vi "USBImageContinuousV1.4.vi"() -> ()   [LabVIEW 2017]
uses:
  C:/Program Files (x86)/National Instruments/LabVIEW 2019/ATMCD32D.dll
  <vilib>/Utility/file.llb/Write Delimited Spreadsheet (I64).vi
  C:/Users/Spenser Burrows/Desktop/Work/Labview software for spectrometer/PiezoStage_John/Piezojena.Protocols.Nv40Single.dll
  E/PiezoStage_John/piezojena NV40Single.lvlib
panel:
  in  "Tab Control":T1(tab)
  out "Expected position on spectrometer (pixels):":dbl
  in  "Harmonic":dbl min=10.0 max=40.0
  out "l (nm)":dbl
  out "E (J)":dbl
  out "E (eV)":dbl
  out "Nearest Harmonic of 800nm":dbl
  out "Cursor Position (pixels)":dbl
  out "Distance to nearest harmonic of 800nm (pixels)":dbl
  in  "Grating:":u16(ring) items=["Shimadzu 30-006  "]
  in  "Laser:":u16(ring) items=["800nm  "]
  in  "Trigger":u32(ring) items=["Internal", "External"]
  out "Initialize":u32
  in  "Exposure Time (secs)":sgl format="%.2f"
  out "Calculated Exposure Value":sgl format="%.5f"
  out "Get Acquired Data":u32
  out "Start Acquisition":u32
  out "Detector X Pixels":i32
  out "Check Timings":u32
  out "Set Acquisition Mode":u32
  out "Set Readout Mode":u32
  out "Set Trigger Mode":u32
  out "Set Exposure Time":u32
  out "Get Detector":u32
  out "Detector Y Pixels":i32
  out "Shut Down":u32
  out "Set Gate Mode":u32
  out "Set Image":u32
  out "Raw Image From Camera":i32[][](graph)
  out "Vertical Binned Waveform Graph":i32[](graph)
  out "Get Status":u32
  in  "Stop":bool
  in  "Save image":bool
  out "Camera Status:":bool
  out "Last Image Saved:":string
  in  "Caibration Date":u16(ring) items=["first calibration - 7/31", "7/31-current"]
  out "Wavelength Graph (nm)":cluster{"No prefix":dbl, i32}[](graph)
  out "Energy Graph (eV)":cluster{"eV":dbl, i32}[](graph)
  out "Harmonics Graph":cluster{"No prefix":dbl, i32}[](graph)
  in  "Measurement Length [fs]":ext=30.0
  out "Optical Cycles \nin measurement":ext=16.905589736842103296
  in  "Initial Piezo Position":sgl=40.0
  out "Number of Steps":ext=300.00000000000005795
  in  "Step Size [as]":sgl=100.0
  in  "?":bool
  in  "Settings":bool
  in  "Wavelength (nm)":i32(listbox)
  in  "Piezojena Seriel Port":refnum<visa-resource-name>="COM4"
  out "Piezo Voltage Supply":cluster{dbl[], dbl[]}(graph)={[0.0], [70.08999633789062]}
  in  "Initial Piezo Position [um]":dbl(slide)=40.0 scale=0.0..80.0
  in  "Final Piezo Position [um]":dbl(slide)=48.99377374 scale=0.0..80.0
  out "Volt Meter":dbl(knob)=70.08999633789062 scale=-10.0..150.0
  out "Raw Image From Camera":i32[][](graph)
  out "Status":u32
  # "Status"
  # "Return values"
  # "Acquisition Mode: Single Scan\nReadout Mode: Full Resolution Image"
  # "XUV Spectrometer Control VI"
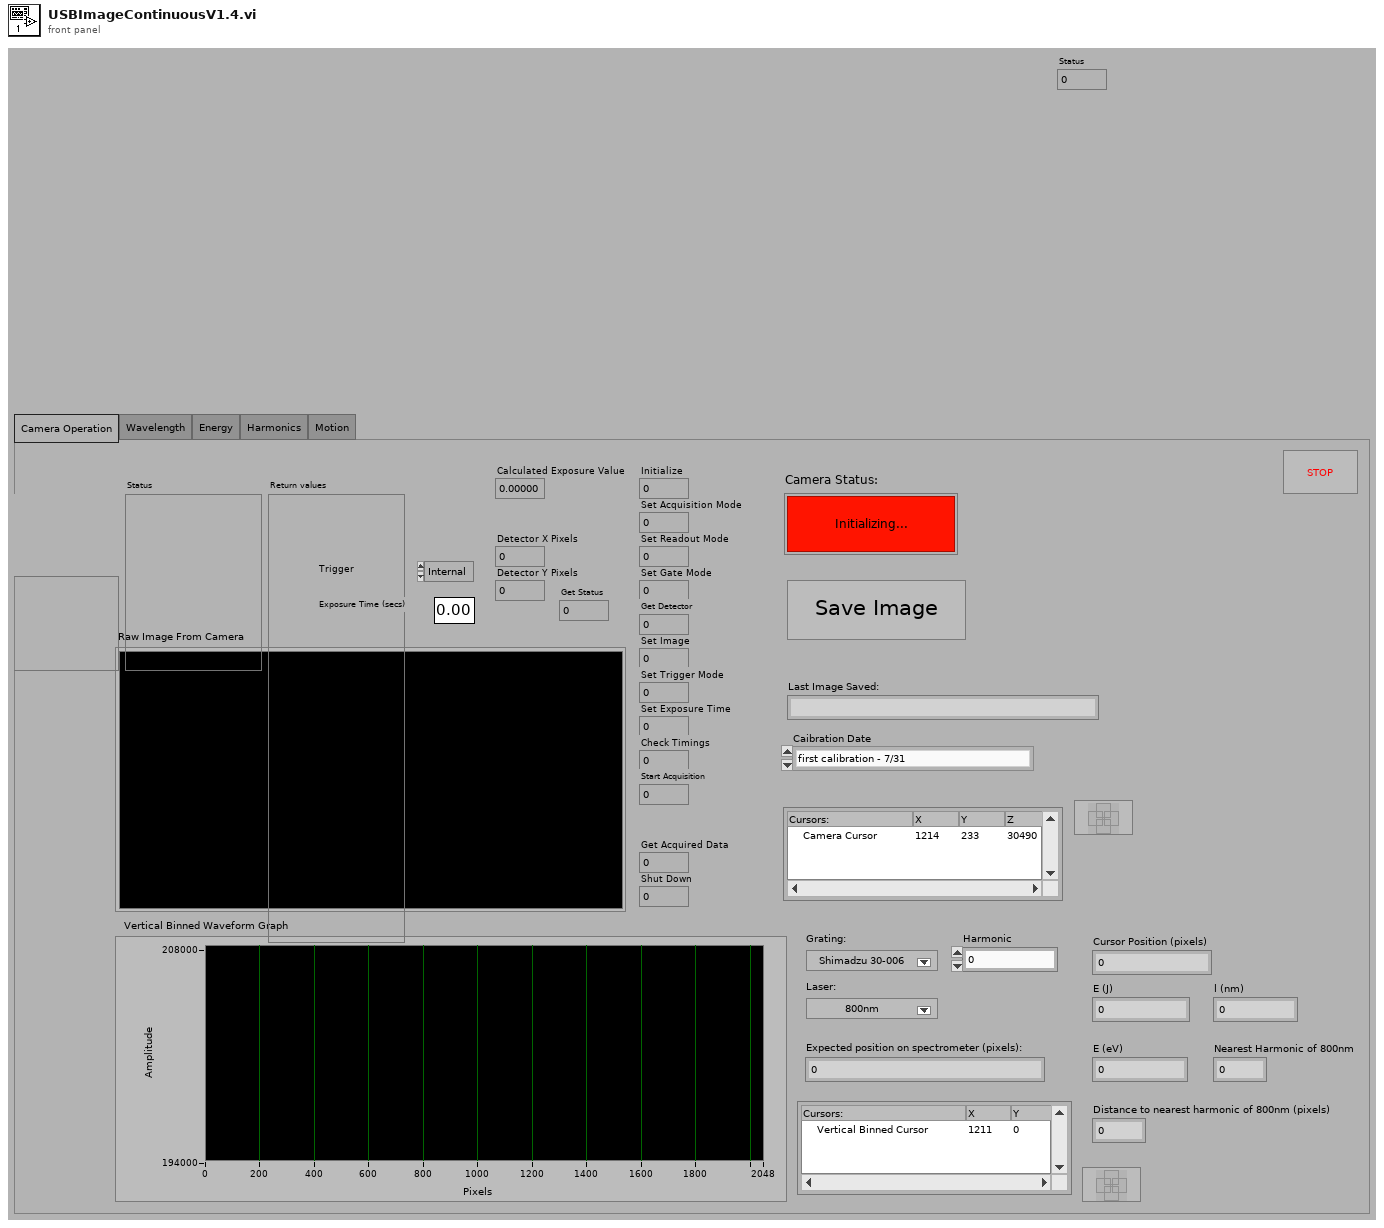
[diagram p1: front panel]
types:
  T1 = enum32{"Camera Operation", "Wavelength", "Energy", "Harmonics", "Motion"}
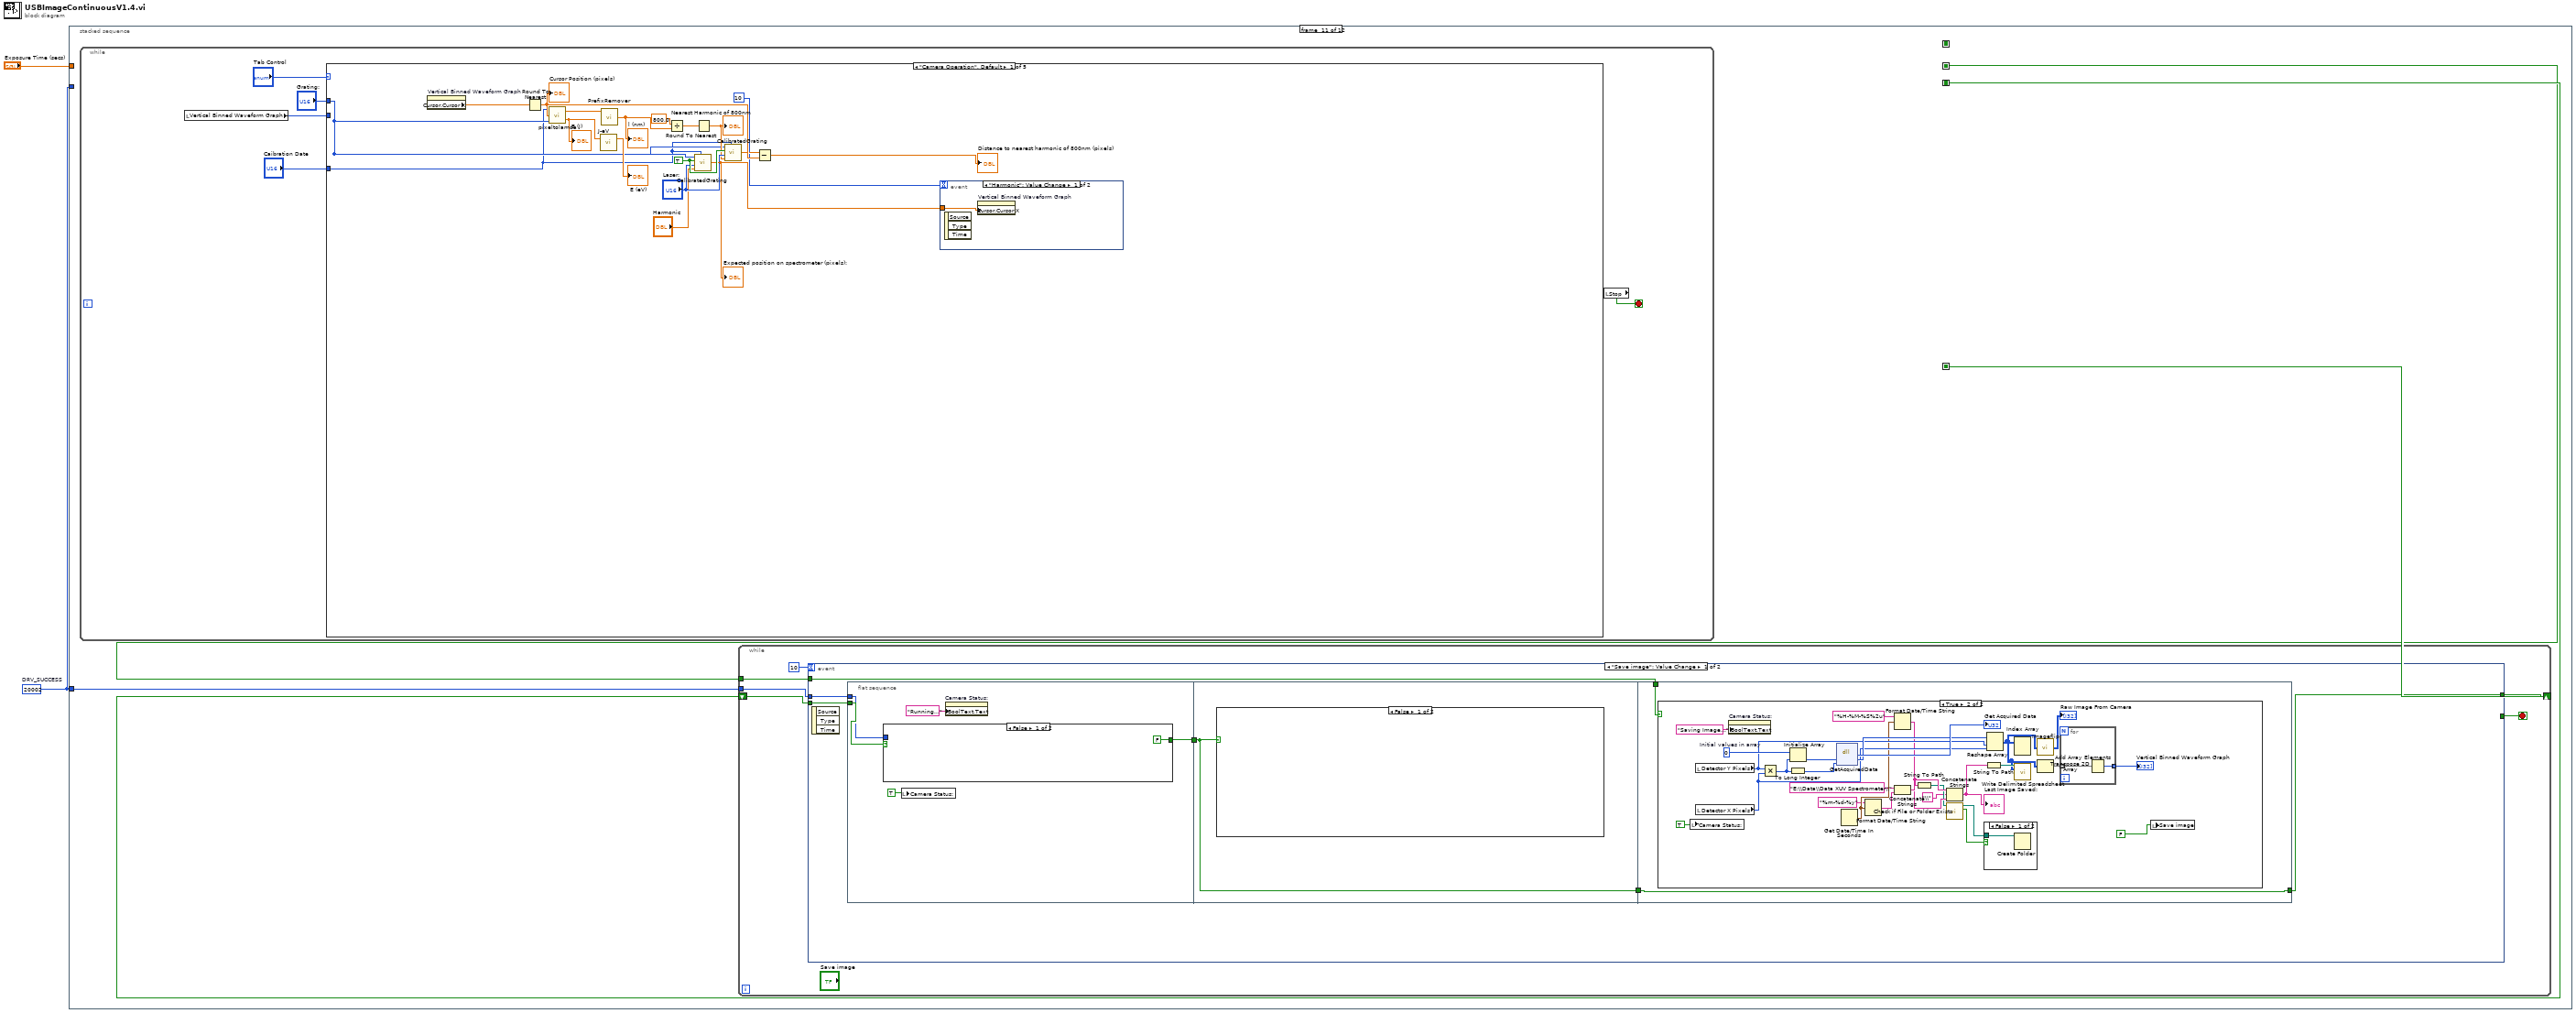
[diagram p0: block diagram]
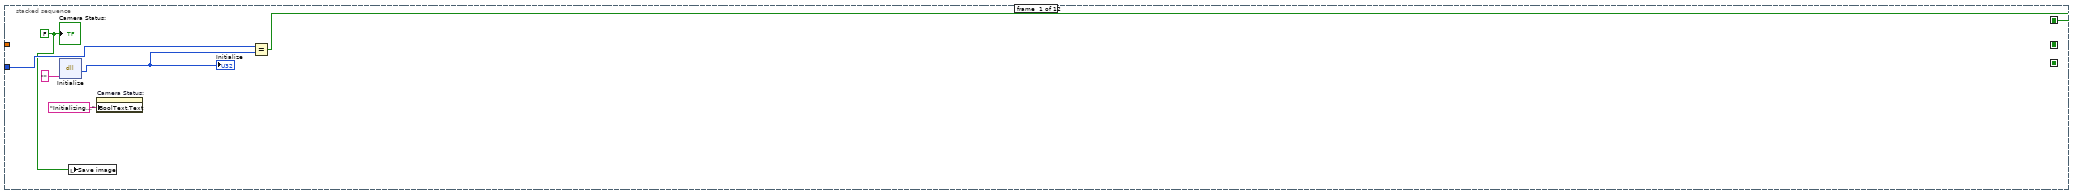
[diagram p2: hidden frame]
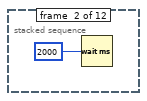
[diagram p3: hidden frame]
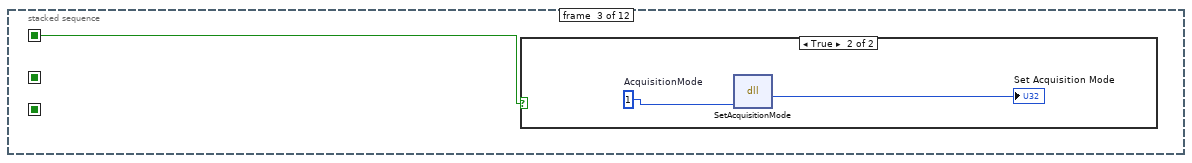
[diagram p4: hidden frame]
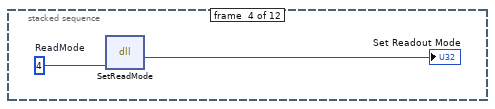
[diagram p6: hidden frame]
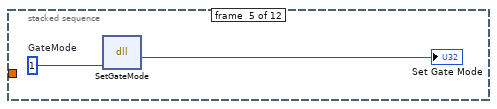
[diagram p7: hidden frame]
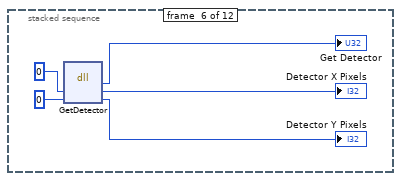
[diagram p8: hidden frame]
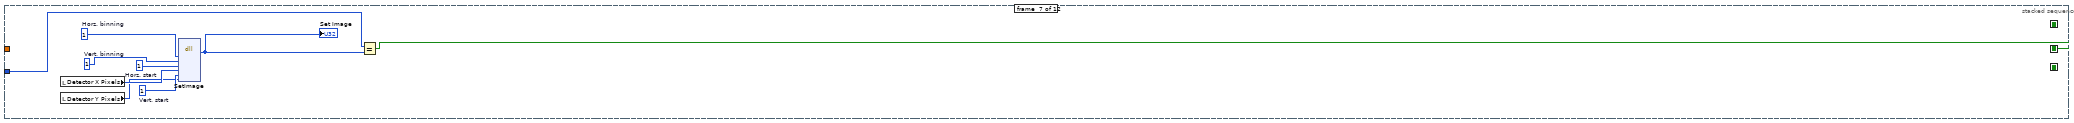
[diagram p9: hidden frame]
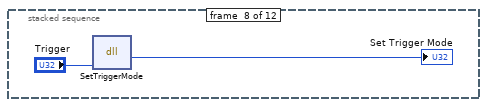
[diagram p10: hidden frame]
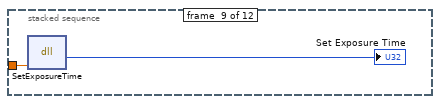
[diagram p11: hidden frame]
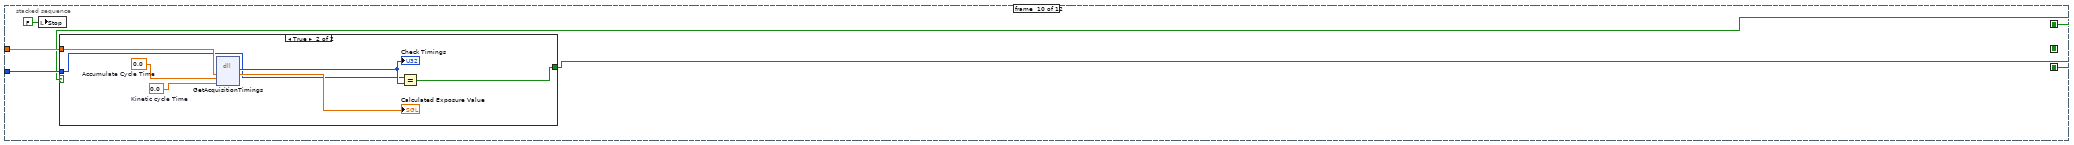
[diagram p12: hidden frame]
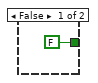
[diagram p13: hidden frame]
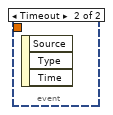
[diagram p14: hidden frame]
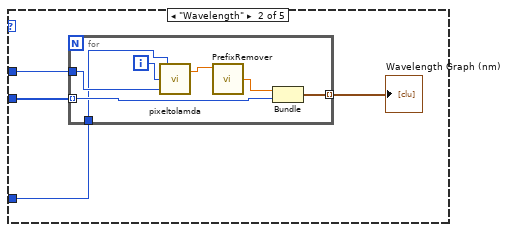
[diagram p15: hidden frame]
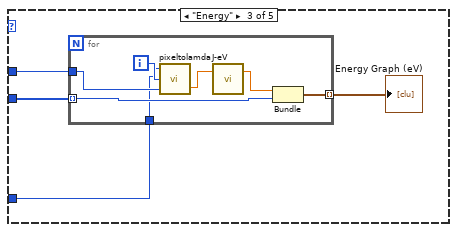
[diagram p16: hidden frame]
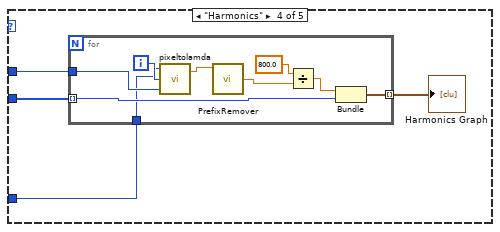
[diagram p17: hidden frame]
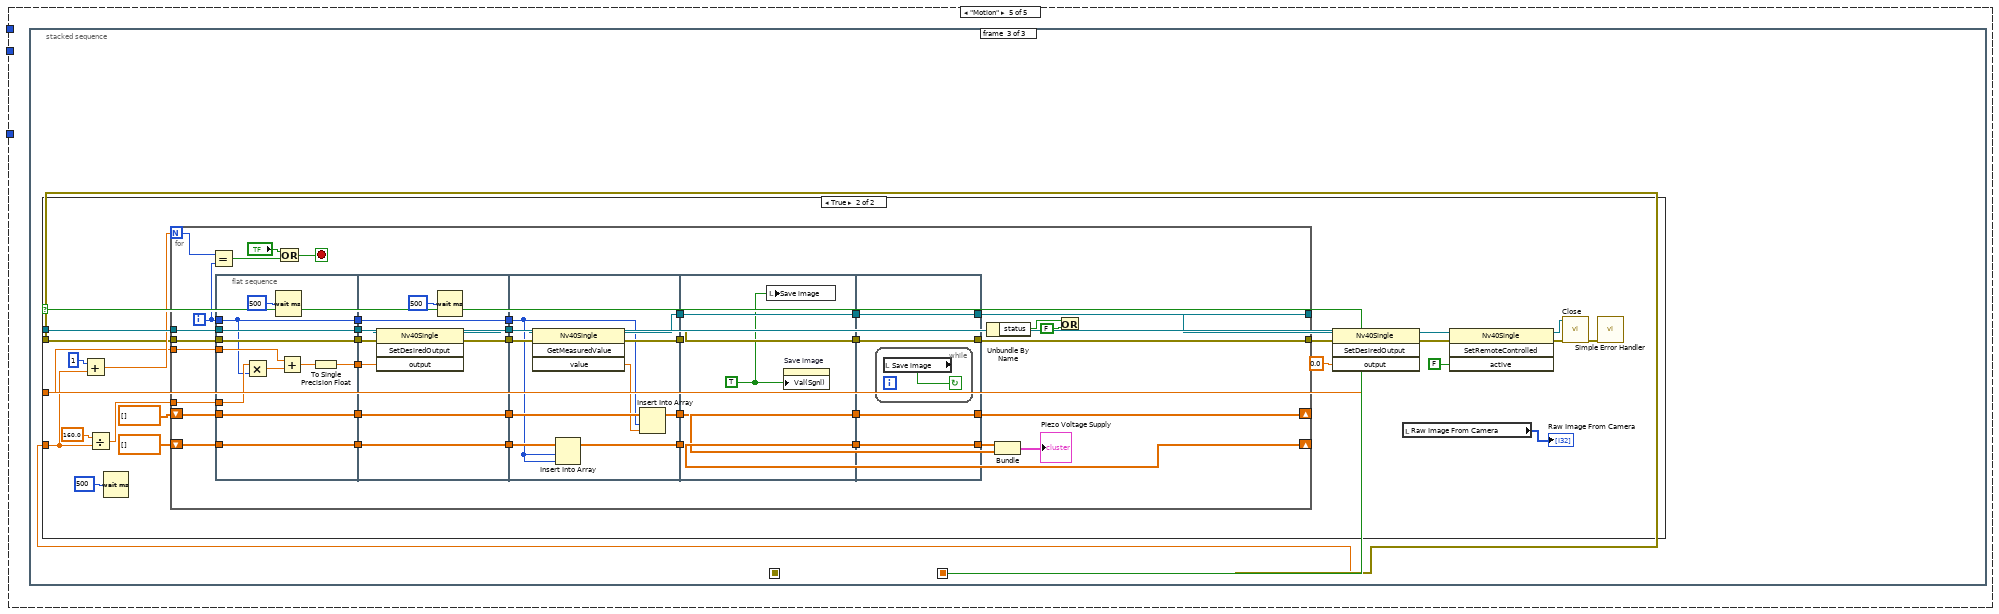
[diagram p18: hidden frame]
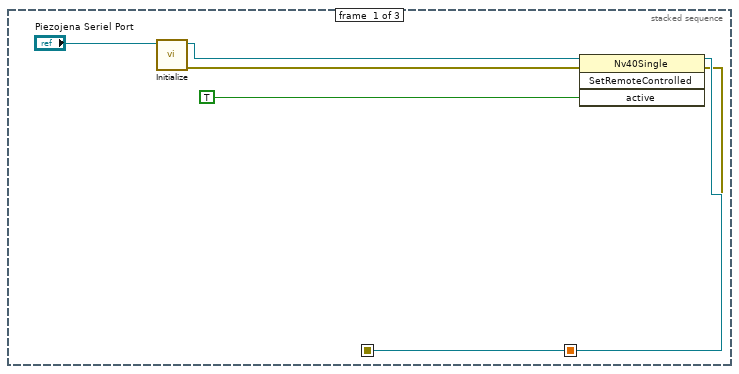
[diagram p19: hidden frame]
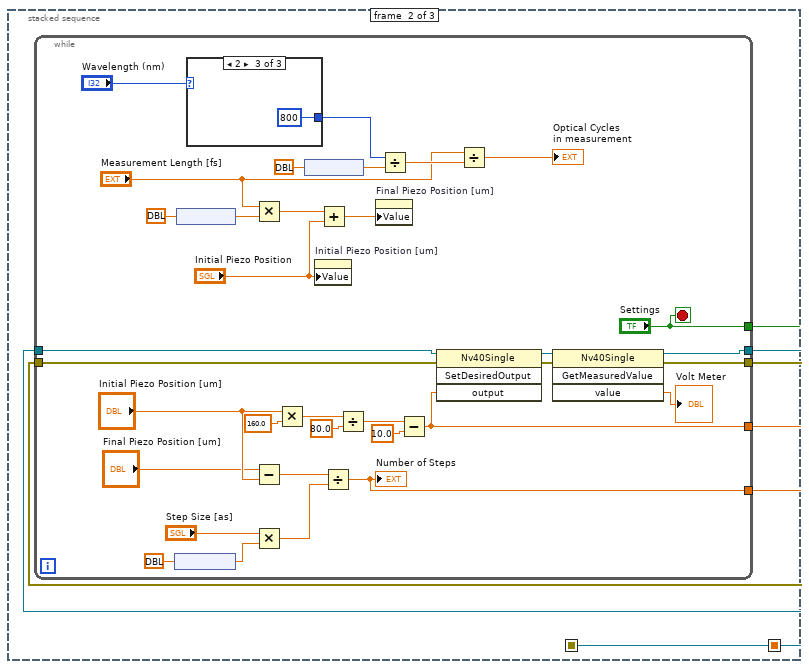
[diagram p20: hidden frame]
diagram:
  w1 = 20002  # DRV_SUCCESS
  n1 = stacked-sequence {
    seq-local: [w6 _ _ _ _ _ _ _ _ _ _ _] -> [_ _ w10 _ _ _ _ _ _ w36 _ w378]
    seq-local: [_ _ _ _ _ _ _ _ _ w37 _ _] -> [_ _ _ _ _ _ _ _ _ _ w51 _]
    seq-local: [_ _ _ _ _ _ _ _ _ _ w49 _] -> [_ _ _ _ _ _ _ _ _ _ _ _]
    seq-local: [_ _ _ _ _ _ w22 _ _ _ _ _] -> [_ _ _ _ _ _ _ _ _ _ w48 _]
    tunnel: "Exposure Time (secs)" -> [_ _ _ _ _ _ _ _ w34 w39 _ _]
    tunnel: w1 -> [w7 _ _ _ _ _ w24 _ _ w38 _ _]
    tunnel: w1 -> [_ _ _ _ _ _ _ _ _ _ w50 _]
    frame #0 {
      w3 = FALSE ("Camera Status:")
      n2 = dll-call lib="C:/Program Files (x86)/National Instruments/LabVIEW 2019/atmcd32d.dll" fn="Initialize" label="Call Library Function Initialize"("") -> (w8:u32)  [unwired: 4 in, 2 out]
      "Initialize" <- w8
      n3 = local write "Save image"(w3) -> ()
      n4 = property on="Camera Status:" class="Bool (strict)"("BoolText.Text"="Initializing..." ("String")) -> ()  [unwired: 2 in, 2 out]
      n5 = Equal?(x=w7, y=w8) -> (x = y?=w6:bool)
      "Camera Status:" <- w3
    }
    frame #1 {
      n6 = Wait (ms)(milliseconds to wait=u32 2000) -> ()  [unwired: 1 out]
    }
    frame #2 {
      n7 = case shown="True" w10 {
        frame False {
        }
        frame True {
          w12 = u16 1  # AcquisitionMode
          n8 = dll-call lib="C:/Program Files (x86)/National Instruments/LabVIEW 2019/atmcd32d.dll" fn="SetAcquisitionMode" label="Call Library Function SetAcquisitionMode"(w12) -> (→"Set Acquisition Mode":u32)  [unwired: 4 in, 2 out]
        }
      }
    }
    frame #3 {
      w14 = u16 4  # ReadMode
      n9 = dll-call lib="C:/Program Files (x86)/National Instruments/LabVIEW 2019/atmcd32d.dll" fn="SetReadMode" label="Call Library Function SetReadMode"(w14) -> (→"Set Readout Mode":u32)  [unwired: 4 in, 2 out]
    }
    frame #4 {
      w16 = u16 1  # GateMode
      n10 = dll-call lib="C:/Program Files (x86)/National Instruments/LabVIEW 2019/atmcd32d.dll" fn="SetGateMode" label="Call Library Function SetGateMode"(w16) -> (→"Set Gate Mode":u32)  [unwired: 4 in, 2 out]
    }
    frame #5 {
      n11 = dll-call lib="C:/Program Files (x86)/National Instruments/LabVIEW 2019/atmcd32d.dll" fn="GetDetector" label="Call Library FunctionGetDetector"(i16 0, i16 0) -> (→"Get Detector":u32, →"Detector X Pixels":i32, →"Detector Y Pixels":i32)  [unwired: 3 in, 2 out]
    }
    frame #6 {
      w27 = u16 1  # Vert. start
      w28 = u16 1  # Horz. start
      w29 = u16 1  # Vert. binning
      w30 = u16 1  # Horz. binning
      n12 = local read "Detector X Pixels"() -> (w26:i32)
      n13 = local read "Detector Y Pixels"() -> (w25:i32)
      n14 = dll-call lib="C:/Program Files (x86)/National Instruments/LabVIEW 2019/atmcd32d.dll" fn="SetImage" label="Call Library Function SetImage"(w30, w29, w28, w26, w27, w25) -> (w23:u32)  [unwired: 9 in, 2 out]
      "Set Image" <- w23
      n15 = Equal?(x=w24, y=w23) -> (x = y?=w22:bool)
    }
    frame #7 {
      n16 = dll-call lib="C:/Program Files (x86)/National Instruments/LabVIEW 2019/atmcd32d.dll" fn="SetTriggerMode" label="Call Library Function SetTrigger Mode"("Trigger") -> (→"Set Trigger Mode":u32)  [unwired: 4 in, 2 out]
    }
    frame #8 {
      n17 = dll-call lib="C:/Program Files (x86)/National Instruments/LabVIEW 2019/atmcd32d.dll" fn="SetExposureTime" label="Call Library FunctionSet Exposure Time"(w34) -> (→"Set Exposure Time":u32)  [unwired: 4 in, 2 out]
    }
    frame #9 {
      n18 = local write "Stop"(FALSE ("Stop")) -> ()
      n19 = case shown="True" w36 {
        tunnel: w39 -> [_ w44]
        tunnel: w38 -> [_ w41]
        tunnel: [FALSE w43] -> w37
        frame False {
        }
        frame True {
          w46 = sgl 0.0  # Accumulate Cycle Time
          w47 = sgl 0.0  # Kinetic cycle Time
          n20 = dll-call lib="C:/Program Files (x86)/National Instruments/LabVIEW 2019/atmcd32d.dll" fn="GetAcquisitionTimings" label="Call Library Function Check Timings"(w44, w46, w47) -> (w42:u32, →"Calculated Exposure Value":sgl)  [unwired: 5 in, 2 out]
          "Check Timings" <- w42
          n21 = Equal?(x=w41, y=w42) -> (x = y?=w43:bool)
        }
      }
    }
    frame #10 {
      n22 = while {
        stop <- w53 stop-if-true
        n23 = local read "Vertical Binned Waveform Graph"() -> (w55:i32[])
        n24 = case shown="\"Camera Operation\", Default" "Tab Control" {
          tunnel: w55 -> [_ w79 w90 w101 _]
          tunnel: "Grating:" -> [w58 w78 w89 w100 _]
          tunnel: "Caibration Date" -> [w57 w76 w87 w98 _]
          frame "Camera Operation", Default {
            w74 = TRUE
            n25 = property on="Vertical Binned Waveform Graph" class="WFGraph (strict)"() -> ("Cursor.Cursor X"=w71:dbl)  [unwired: 2 in, 2 out]
            n26 = Round To Nearest(number=w71) -> (nearest integer value=w64:dbl)
            "Cursor Position (pixels)" <- w64
            n27 = call "pixeltolamda.vi"("Grating:"=w58, "Pixel Postion"=w64, "Caibration Date"=w57) -> ("E (J)"=w66:dbl, "lamda (m)"=w72:dbl)
            "E (J)" <- w66
            n28 = call "J-eV.vi"("J"=w66) -> ("eV"=→"E (eV)":dbl)  [unwired: 1 in, 1 out]
            n29 = call "PrefixRemover.vi"("Nano"=w72) -> ("No prefix"=w67:dbl)  [unwired: 3 in]
            "l (nm)" <- w67
            n30 = Divide(x=800.0, y=w67) -> (x/y=w69:dbl)
            n31 = call "CalibratedGrating.vi"("Grating:"=w58, "Subvi?"=w74, "Laser:"="Laser:", "Harmonic"="Harmonic", "Caibration Date"=w57) -> ("Position on spectrometer (pixels):"=w60:dbl)
            "Expected position on spectrometer (pixels):" <- w60
            n32 = Round To Nearest(number=w69) -> (nearest integer value=w63:dbl)
            "Nearest Harmonic of 800nm" <- w63
            n33 = call "CalibratedGrating.vi"("Grating:"=w58, "Subvi?"=w74, "Laser:"="Laser:", "Harmonic"=w63, "Caibration Date"=w57) -> ("Position on spectrometer (pixels):"=w62:dbl)
            n34 = Subtract(x=w62, y=w64) -> (x-y=→"Distance to nearest harmonic of 800nm (pixels)":dbl)
            n35 = event shown="[0] \"Harmonic\": Value Change" {
              selector: _ -> [_ _]
              dyn-events: _ -> [_ _]
              timeout: 10 -> [_ _]
              tunnel: w60 -> [w75 _]
              event "Harmonic": Value Change {
                n36 = event-data() -> ()  [unwired: 1 in, 3 out]
                n37 = property on="Vertical Binned Waveform Graph" class="WFGraph (strict)"("Cursor.Cursor X"=w75) -> ()  [unwired: 2 in, 2 out]
              }
              event Timeout {
                n38 = event-data() -> ()  [unwired: 1 in, 3 out]
              }
            }
          }
          frame "Wavelength" {
            n39 = for {
              tunnel: w79 -> [w82] mode=indexing
              tunnel: w78 -> [w84]
              tunnel: [w81] -> w77 mode=indexing
              tunnel: w76 -> [w80]
              i -> [w83]
              n40 = call "pixeltolamda.vi"("Grating:"=w84, "Pixel Postion"=w83, "Caibration Date"=w80) -> ("lamda (m)"=w85:dbl)  [unwired: 1 out]
              n41 = call "PrefixRemover.vi"("Nano"=w85) -> ("No prefix"=w86:dbl)  [unwired: 3 in]
              n42 = Bundle("No prefix"=w86, w82) -> (w81:cluster{"No prefix":dbl, i32})  [unwired: 1 in]
            }
            "Wavelength Graph (nm)" <- w77
          }
          frame "Energy" {
            n43 = for {
              tunnel: w90 -> [w93] mode=indexing
              tunnel: w89 -> [w96]
              tunnel: [w92] -> w88 mode=indexing
              tunnel: w87 -> [w91]
              i -> [w97]
              n44 = call "pixeltolamda.vi"("Grating:"=w96, "Pixel Postion"=w97, "Caibration Date"=w91) -> ("E (J)"=w95:dbl)  [unwired: 1 out]
              n45 = call "J-eV.vi"("J"=w95) -> ("eV"=w94:dbl)  [unwired: 1 in, 1 out]
              n46 = Bundle("eV"=w94, w93) -> (w92:cluster{"eV":dbl, i32})  [unwired: 1 in]
            }
            "Energy Graph (eV)" <- w88
          }
          frame "Harmonics" {
            n47 = for {
              tunnel: w101 -> [w107] mode=indexing
              tunnel: w100 -> [w109]
              tunnel: [w106] -> w99 mode=indexing
              tunnel: w98 -> [w102]
              i -> [w108]
              n48 = call "pixeltolamda.vi"("Grating:"=w109, "Pixel Postion"=w108, "Caibration Date"=w102) -> ("lamda (m)"=w110:dbl)  [unwired: 1 out]
              n49 = call "PrefixRemover.vi"("Nano"=w110) -> ("No prefix"=w104:dbl)  [unwired: 3 in]
              n50 = Divide(x=800.0, y=w104) -> (x/y=w103:dbl)
              n51 = Bundle(w103, w107) -> (w106:cluster{dbl, i32})  [unwired: 1 in]
            }
            "Harmonics Graph" <- w99
          }
          frame "Motion" {
            n52 = stacked-sequence {
              seq-local: [w112 _ _] -> [_ w123 _]
              seq-local: [w111 _ _] -> [_ w122 _]
              seq-local: [_ w121 _] -> [_ _ w165]
              seq-local: [_ w120 _] -> [_ _ w164]
              seq-local: [_ w119 _] -> [_ _ w163]
              seq-local: [_ w118 _] -> [_ _ w162]
              seq-local: [_ w117 _] -> [_ _ w161]
              frame #0 {
                n53 = call "Initialize.vi"("VISA resource name"="Piezojena Seriel Port") -> ("error out"=w116:errorcluster, "Piezojena.Protocols.Nv40Single.Nv40Single"=w115:refnum<k24>)  [unwired: 9 in]
                n54 = invoke class="Nv40Single" method="SetRemoteControlled"(reference=w115, error in=w116, "active"=TRUE) -> (reference out=w112:refnum<k24>, error out=w111:errorcluster)  [unwired: 1 in, 2 out]
              }
              frame #1 {
                n55 = while {
                  tunnel: ["Settings"] -> w121
                  tunnel: [w144] -> w120
                  tunnel: [w156] -> w119
                  tunnel: [w155] -> w118
                  tunnel: w123 -> [w154]
                  tunnel: w122 -> [w153]
                  tunnel: [w138] -> w117
                  stop <- "Settings" stop-if-true
                  n56 = node(ext[unit] 299792458.0) -> (w142:ext)
                  n57 = node(ext[unit] 299792458.0) -> (w129:ext)
                  n58 = case shown="2" "Wavelength (nm)" {
                    tunnel: [532 ("Numeric 2") 633 ("Numeric 2") 800 ("Numeric 2")] -> w133
                    frame 0, Default {
                    }
                    frame 1 {
                    }
                    frame 2 {
                    }
                  }
                  n59 = Multiply(x="Measurement Length [fs]", y=w129) -> (x*y=w127:ext)
                  n60 = Subtract(x="Final Piezo Position [um]", y="Initial Piezo Position [um]") -> (x-y=w141:dbl)
                  n61 = Multiply(x="Step Size [as]", y=w142) -> (x*y=w140:ext)
                  n62 = Multiply(x="Initial Piezo Position [um]", y=160.0 ("x")) -> (x*y=w147:dbl)
                  n63 = node(ext[unit] 299792458.0) -> (w132:ext)
                  n64 = property on="Initial Piezo Position [um]" class="Slide (strict)"("Value"="Initial Piezo Position") -> ()  [unwired: 2 in, 2 out]
                  n65 = Add(x=w127, y="Initial Piezo Position") -> (x+y=w126:ext)
                  n66 = Divide(x=w141, y=w140) -> (x/y=w138:ext)
                  "Number of Steps" <- w138
                  n67 = Divide(x=w147, y=80.0) -> (x/y=w146:dbl)
                  n68 = property on="Final Piezo Position [um]" class="Slide (strict)"("Value"=w126) -> ()  [unwired: 2 in, 2 out]
                  n69 = Divide(x=w133, y=w132) -> (x/y=w125:ext)
                  n70 = Subtract(x=w146, y=10.0) -> (x-y=w144:dbl)
                  n71 = invoke class="Nv40Single" method="SetDesiredOutput"(reference=w154, error in=w153, "output"=w144) -> (reference out=w150:refnum<k24>, error out=w151:errorcluster)  [unwired: 1 in, 2 out]
                  n72 = Divide(x="Measurement Length [fs]", y=w125) -> (x/y=→"Optical Cycles \nin measurement":ext)
                  n73 = invoke class="Nv40Single" method="GetMeasuredValue"(reference=w150, error in=w151) -> (reference out=w156:refnum<k24>, error out=w155:errorcluster, "value"=→"Volt Meter":sgl)  [unwired: 2 in, 1 out]
                }
              }
              frame #2 {
                n74 = case shown="True" w165 {
                  tunnel: w164 -> [_ w179]
                  tunnel: w163 -> [_ w178]
                  tunnel: w162 -> [_ w177]
                  tunnel: w161 -> [_ w173]
                  frame False {
                    (unwired) TRUE ("Stop Measurement 2")
                  }
                  frame True {
                    n75 = Add(x=1 ("y"), y=w173) -> (x+y=w180:ext)
                    n76 = Divide(x=160.0, y=w173) -> (x/y=w172:ext)
                    n77 = Wait (ms)(milliseconds to wait=u32 500 ("Wait for \nPiezo to start 2")) -> ()  [unwired: 1 out]
                    n78 = for {
                      N: w180 -> [w221]
                      tunnel: [w223] -> w171
                      tunnel: [w222] -> w170
                      tunnel: w178 -> [w213]
                      tunnel: w177 -> [w212]
                      tunnel: w179 -> [w208]
                      shift-right: [w196] -> _
                      shift-left: dbl[] [] -> [w206]
                      shift-right: [w197] -> _
                      shift-left: dbl[] [] -> [w201]
                      tunnel: w172 -> [w195]
                      i -> [w207]
                      stop <- w220 stop-if-true
                      n79 = Equal?(x=w221, y=w207) -> (x = y?=w219:bool)
                      n80 = flat-sequence {
                        tunnel: w212 -> [w233]
                        tunnel: w213 -> [w234]
                        tunnel: [w234] -> w211
                        tunnel: [w233] -> w210
                        tunnel: [w229] -> w209
                        tunnel: w207 -> [w226]
                        tunnel: w195 -> [w231]
                        tunnel: w208 -> [w230]
                        tunnel: w206 -> [w227]
                        tunnel: [w227] -> w205
                        tunnel: [w226] -> w202
                        tunnel: w201 -> [w224]
                        tunnel: [w224] -> w200
                        tunnel: [w239] -> w217
                        tunnel: [w238] -> w216
                        tunnel: w211 -> [w242]
                        tunnel: w210 -> [w241]
                        tunnel: w209 -> [w240]
                        tunnel: w205 -> [w237]
                        tunnel: [w237] -> w204
                        tunnel: [w236] -> w203
                        tunnel: w202 -> [w236]
                        tunnel: w200 -> [w235]
                        tunnel: [w235] -> w199
                        tunnel: w217 -> [w250]
                        tunnel: w216 -> [w249]
                        tunnel: w204 -> [w248]
                        tunnel: w203 -> [w245]
                        tunnel: w199 -> [w246]
                        tunnel: [w253] -> w194
                        tunnel: [w252] -> w193
                        tunnel: [w251] -> w192
                        tunnel: [w247] -> w191
                        tunnel: w194 -> [w258]
                        tunnel: w193 -> [w257]
                        tunnel: w192 -> [w256]
                        tunnel: w191 -> [w255]
                        tunnel: [w258] -> w190
                        tunnel: [w257] -> w189
                        tunnel: [w256] -> w188
                        tunnel: [w255] -> w187
                        tunnel: [w259] -> w197
                        tunnel: [w260] -> w196
                        tunnel: [w261] -> w222
                        tunnel: [w262] -> w223
                        tunnel: w190 -> [w262]
                        tunnel: w189 -> [w261]
                        tunnel: w188 -> [w260]
                        tunnel: w187 -> [w259]
                        frame #0 {
                          n81 = Multiply(x=w231, y=w226) -> (x*y=w225:ext)
                          n82 = Wait (ms)(milliseconds to wait=u32 500 ("Delay (ms) 3")) -> ()  [unwired: 1 out]
                          n83 = Add(x=w230, y=w225) -> (x+y=w232:ext)
                          n84 = To Single Precision Float(number=w232) -> (single precision float=w229:sgl)
                        }
                        frame #1 {
                          n85 = invoke class="Nv40Single" method="SetDesiredOutput"(reference=w242, error in=w241, "output"=w240) -> (reference out=w239:refnum<k24>, error out=w238:errorcluster)  [unwired: 1 in, 2 out]
                          n86 = Wait (ms)(milliseconds to wait=u32 500 ("Delay (ms) 4")) -> ()  [unwired: 1 out]
                        }
                        frame #2 {
                          n87 = invoke class="Nv40Single" method="GetMeasuredValue"(reference=w250, error in=w249) -> (reference out=w253:refnum<k24>, error out=w252:errorcluster, "value"=w244:sgl)  [unwired: 2 in, 1 out]
                          n88 = Insert Into Array(array=w246, index=w245, new element=w245) -> (w247:dbl[])
                          n89 = Insert Into Array(array=w248, index=w245, new element=w244) -> (w251:dbl[])
                        }
                        frame #3 {
                          w254 = TRUE
                          n90 = local write "Save image"(w254) -> ()
                          n91 = property on="Save image" class="Bool (strict)"("Val(Sgnl)"=w254) -> ()  [unwired: 2 in, 2 out]
                        }
                        frame #4 {
                          n92 = while {
                            stop <- w263 continue-if-true
                            n93 = local read "Save image"() -> (w263:bool)
                          }
                        }
                      }
                      n94 = Or(x="?", y=w219) -> (x .or. y?=w220:bool)
                      n95 = Unbundle By Name(w222) -> ("status"=w215:bool)
                      n96 = Bundle(w197, w196) -> (→"Piezo Voltage Supply":cluster{dbl[], dbl[]})  [unwired: 1 in]
                      n97 = Or(x=w215, y=FALSE ("Halt Measurment")) -> ()  [unwired: 1 out]
                    }
                    n98 = invoke class="Nv40Single" method="SetDesiredOutput"(reference=w171, error in=w170, "output"=sgl 0.0) -> (reference out=w168:refnum<k24>, error out=w167:errorcluster)  [unwired: 1 in, 2 out]
                    n99 = local read "Raw Image From Camera"() -> (→"Raw Image From Camera":i32[][])
                    n100 = invoke class="Nv40Single" method="SetRemoteControlled"(reference=w168, error in=w167, "active"=FALSE) -> (reference out=w185:refnum<k24>, error out=w183:errorcluster)  [unwired: 1 in, 2 out]
                    n101 = call "Close.vi"("error in (no error)"=w183, "reference"=w185) -> ("error out"=w186:errorcluster)  [unwired: 9 in]
                    n102 = call <vilib>:"Simple Error Handler.vi"("error in (no error)"=w186) -> ()  [unwired: 4 in, 5 out]
                  }
                }
              }
            }
          }
        }
        n103 = local read "Stop"() -> (w53:bool)
      }
      n104 = while {
        tunnel: w50 -> [w268]
        tunnel: w48 -> [w266]
        shift-right: [w267] -> w49
        shift-left: w51 -> [w269]
        stop <- w264 stop-if-true
        n105 = event shown="[0] \"Save image\": Value Change" {
          selector: _ -> [_ _]
          dyn-events: _ -> [_ _]
          timeout: 10 -> [_ _]
          tunnel: w269 -> [w273 w330]
          tunnel: w268 -> [w272 w329]
          tunnel: [w271 w328] -> w267
          tunnel: w266 -> [w270 w327]
          tunnel: [_ w326] -> w264
          event "Save image": Value Change {
            n106 = event-data() -> ()  [unwired: 1 in, 3 out]
            n107 = flat-sequence {
              tunnel: w273 -> [w280]
              tunnel: w272 -> [w279]
              tunnel: [w278] -> w275
              tunnel: w275 -> [w285]
              tunnel: [w285] -> w274
              tunnel: [w293] -> w271
              tunnel: w274 -> [w293]
              tunnel: w270 -> [w292]
              frame #0 {
                n108 = case shown="False" w280 {
                  tunnel: [FALSE w283] -> w278
                  tunnel: w279 -> [_ w282]
                  frame False {
                  }
                  frame True {
                    n109 = dll-call lib="C:/Program Files (x86)/National Instruments/LabVIEW 2019/atmcd32d.dll" fn="StartAcquisition" label="Call Library Function start acquisition"() -> (w284:u32)  [unwired: 3 in, 2 out]
                    "Start Acquisition" <- w284
                    n110 = Equal?(x=w282, y=w284) -> (x = y?=w283:bool)
                  }
                }
                n111 = local write "Camera Status:"(TRUE ("Camera Status:")) -> ()
                n112 = property on="Camera Status:" class="Bool (strict)"("BoolText.Text"="Running..." ("Boolean Text.Text")) -> ()  [unwired: 2 in, 2 out]
              }
              frame #1 {
                n113 = case shown="False" w285 {
                  frame False {
                  }
                  frame True {
                    n114 = while {
                      stop <- w289 continue-if-true
                      w288 = u16 20072  # DRV ACQUIRING
                      n115 = Wait Until Next ms Multiple(millisecond multiple=u32 500) -> ()  [unwired: 1 out]
                      n116 = dll-call lib="C:/Program Files (x86)/National Instruments/LabVIEW 2019/atmcd32d.dll" fn="GetStatus" label="Call Library Function GetAcquisitionStatus"(u16 0) -> (→"Get Status":u32, w287:u32)  [unwired: 3 in, 2 out]
                      "Status" <- w287
                      n117 = Equal?(x=w287, y=w288) -> (x = y?=w289:bool)
                    }
                  }
                }
              }
              frame #2 {
                n118 = case shown="True" w292 {
                  frame False {
                  }
                  frame True {
                    w321 = 0  # Initial values in array
                    n119 = local write "Camera Status:"(TRUE ("Camera Status:")) -> ()
                    n120 = local read "Detector Y Pixels"() -> (w315:i32)
                    n121 = local read "Detector X Pixels"() -> (w314:i32)
                    n122 = property on="Camera Status:" class="Bool (strict)"("BoolText.Text"="Saving Image..." ("Boolean Text.Text")) -> ()  [unwired: 2 in, 2 out]
                    n123 = Multiply(x=w315, y=w314) -> (x*y=w317:i32)
                    n124 = To Long Integer(number=w317) -> (32bit integer=w318:i32)
                    n125 = Initialize Array "Initialize Array"(w321, w317) -> (w319:i32[])
                    n126 = dll-call lib="C:/Program Files (x86)/National Instruments/LabVIEW 2019/atmcd32d.dll" fn="GetAcquiredData" label="Call Library Function Get Acquired data"(w319, w318) -> (→"Get Acquired Data":u32, w316:i32[])  [unwired: 4 in, 2 out]
                    n127 = Get Date/Time In Seconds() -> (seconds since 1Jan1904=w311:timestamp)
                    n128 = Format Date/Time String(time format string (%c)="%m-%d-%y", seconds (now)=w311) -> (date/time string=w309:string)  [unwired: 1 in]
                    n129 = Format Date/Time String(time format string (%c)="%H-%M-%S%2u", seconds (now)=w311) -> (date/time string=w310:string)  [unwired: 1 in]
                    n130 = Concatenate Strings("E:\\Data\\Data XUV Spectrometer\\" ("string"), w309) -> (w312:string)
                    n131 = String To Path(string=w312) -> (path=w308:path)
                    n132 = Concatenate Strings(w312, "\\" ("string"), w310) -> (w313:string)
                    "Last Image Saved:" <- w313
                    n133 = call <vilib>:"Check if File or Folder Exists.vi"("path"=w308) -> ("file or folder exists?"=w306:bool, "dup path"=w307:path)  [unwired: 8 in, 1 out]
                    n134 = case shown="False" w306 {
                      tunnel: w307 -> [w324 _]
                      frame False {
                        n135 = Create Folder(path (use dialog)=w324) -> ()  [unwired: 2 in, 3 out]
                      }
                      frame True {
                      }
                    }
                    n136 = String To Path(string=w313) -> (path=w301:path)
                    n137 = Reshape Array(w316, w315, w314) -> (w296:i32[][])
                    n138 = Index Array(array=w296) -> ()  [unwired: 2 in, 1 out]
                    n139 = call-poly <vilib>:"Write Delimited Spreadsheet.vi"("file path (dialog if empty)"=w301, "2D data"=w296) -> ()  [unwired: 12 in, 2 out]
                    n140 = call "Imageflip.vi"("2D array"=w296) -> ("transposed array"=→"Raw Image From Camera":i32[][])
                    n141 = Transpose 2D Array(2D array=w296) -> (transposed array=w300:i32[][])
                    n142 = for {
                      tunnel: w300 -> [w323] mode=indexing
                      tunnel: [w322] -> w299 mode=indexing
                      n143 = Add Array Elements(numeric array=w323) -> (sum=w322:i32)
                    }
                    "Vertical Binned Waveform Graph" <- w299
                    n144 = local write "Save image"(FALSE ("Take image")) -> ()
                  }
                }
              }
            }
          }
          event Timeout {
            n145 = event-data() -> ()  [unwired: 1 in, 3 out]
            n146 = flat-sequence {
              tunnel: w330 -> [w337]
              tunnel: w329 -> [w336]
              tunnel: [w335] -> w332
              tunnel: w332 -> [w342]
              tunnel: [w342] -> w331
              tunnel: w331 -> [w349]
              tunnel: w327 -> [w350]
              tunnel: [w349] -> w325
              tunnel: ["Stop"] -> w326
              tunnel: [w375] -> w328
              tunnel: w325 -> [w375]
              frame #0 {
                n147 = case shown="True" w337 {
                  tunnel: [FALSE w341] -> w335
                  tunnel: w336 -> [_ w340]
                  frame False {
                  }
                  frame True {
                    n148 = dll-call lib="C:/Program Files (x86)/National Instruments/LabVIEW 2019/atmcd32d.dll" fn="StartAcquisition" label="Call Library Function start acquisition"() -> (w339:u32)  [unwired: 3 in, 2 out]
                    n149 = local write "Start Acquisition"(w339) -> ()
                    n150 = Equal?(x=w340, y=w339) -> (x = y?=w341:bool)
                  }
                }
                n151 = local write "Camera Status:"(TRUE ("Camera Status:")) -> ()
                n152 = property on="Camera Status:" class="Bool (strict)"("BoolText.Text"="Running..." ("Boolean Text.Text")) -> ()  [unwired: 2 in, 2 out]
              }
              frame #1 {
                n153 = case shown="True" w342 {
                  frame False {
                  }
                  frame True {
                    n154 = while {
                      stop <- w346 continue-if-true
                      w345 = u16 20072  # DRV ACQUIRING
                      n155 = Wait Until Next ms Multiple(millisecond multiple=u32 500) -> ()  [unwired: 1 out]
                      n156 = dll-call lib="C:/Program Files (x86)/National Instruments/LabVIEW 2019/atmcd32d.dll" fn="GetStatus" label="Call Library Function GetAcquisitionStatus"(u16 0) -> (w344:u32, w343:u32)  [unwired: 3 in, 2 out]
                      n157 = local write "Status"(w343) -> ()
                      n158 = local write "Get Status"(w344) -> ()
                      n159 = Equal?(x=w343, y=w345) -> (x = y?=w346:bool)
                    }
                  }
                }
              }
              frame #2 {
                n160 = case shown="True" w350 {
                  frame False {
                  }
                  frame True {
                    w365 = 0  # Initial values in array
                    n161 = local read "Detector Y Pixels"() -> (w360:i32)
                    n162 = local read "Detector X Pixels"() -> (w359:i32)
                    n163 = Multiply(x=w360, y=w359) -> (x*y=w362:i32)
                    n164 = Initialize Array "Initialize Array"(w365, w362) -> (w364:i32[])
                    n165 = To Long Integer(number=w362) -> (32bit integer=w363:i32)
                    n166 = dll-call lib="C:/Program Files (x86)/National Instruments/LabVIEW 2019/atmcd32d.dll" fn="GetAcquiredData" label="Call Library Function Get Acquired data"(w364, w363) -> (w357:u32, w361:i32[])  [unwired: 4 in, 2 out]
                    n167 = local write "Get Acquired Data"(w357) -> ()
                    n168 = Reshape Array(w361, w360, w359) -> (w351:i32[][])
                    n169 = Index Array(array=w351) -> ()  [unwired: 2 in, 1 out]
                    n170 = Array Max & Min(array=w351) -> (max value=w355:i32)  [unwired: 3 out]
                    n171 = Transpose 2D Array(2D array=w351) -> (transposed array=w358:i32[][])
                    n172 = call "Imageflip.vi"("2D array"=w351) -> ("transposed array"=w352:i32[][])
                    n173 = local write "Raw Image From Camera"(w352) -> ()
                    n174 = for {
                      tunnel: w358 -> [w373] mode=indexing
                      tunnel: [w372] -> w356 mode=indexing
                      n175 = Add Array Elements(numeric array=w373) -> (sum=w372:i32)
                    }
                    n176 = Greater?(x=w355, y=64900) -> (0:w353:bool)
                    n177 = case shown="True" w353 {
                      frame False {
                      }
                      frame True {
                        n178 = local write "Camera Status:"(FALSE ("Camera Status:")) -> ()
                        n179 = property on="Camera Status:" class="Bool (strict)"("BoolText.Text"="Saturated!" ("Boolean Text.Text")) -> ()  [unwired: 2 in, 2 out]
                        n180 = Two Button Dialog(message="Camera is saturating! Reduce photon flux!", 1:"I've fixed it, and I want to continue" ("message"), 2:"Shut Down Camera" ("T button name (\"OK\")")) -> (T button?=w367:bool)
                        n181 = local write "Stop"(w367) -> ()
                      }
                    }
                    n182 = local write "Vertical Binned Waveform Graph"(w356) -> ()
                  }
                }
              }
              frame #3 {
              }
            }
          }
        }
      }
    }
    frame #11 {
      n183 = local write "Camera Status:"(FALSE ("Camera Status:")) -> ()
      n184 = property on="Camera Status:" class="Bool (strict)"("BoolText.Text"="Shutting Down..." ("Boolean Text.Text")) -> ()  [unwired: 2 in, 2 out]
      n185 = case shown="True" w378 {
        frame False {
        }
        frame True {
          n186 = dll-call lib="C:/Program Files (x86)/National Instruments/LabVIEW 2019/atmcd32d.dll" fn="ShutDown" label="Call Library Function Shutdown"() -> (→"Shut Down":u32)  [unwired: 3 in, 2 out]
        }
      }
    }
  }
